vi "testserialRT.vi"() -> ()   [LabVIEW 2017]
uses:
  <vilib>/Instr/_visa.llb/VISA Configure Serial Port (Instr).vi
panel:
  out "error out":errorcluster
  out "s? t:f":i32
  out "4":dbl
  out "3":dbl
  out "2":dbl
  out "1":dbl
  out "Fy":dbl
  out "Fx":dbl
  out "String":string
  in  "stop":bool
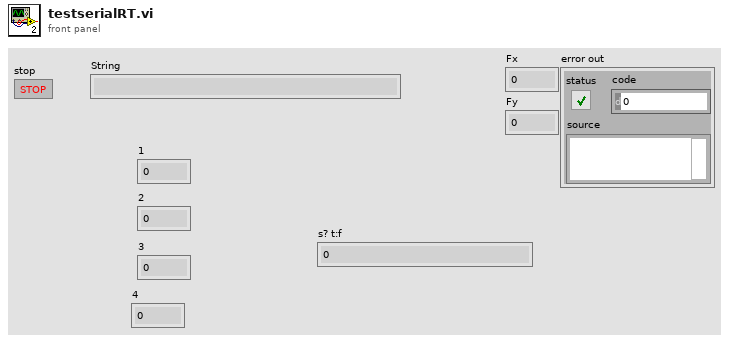
[diagram p1: front panel]
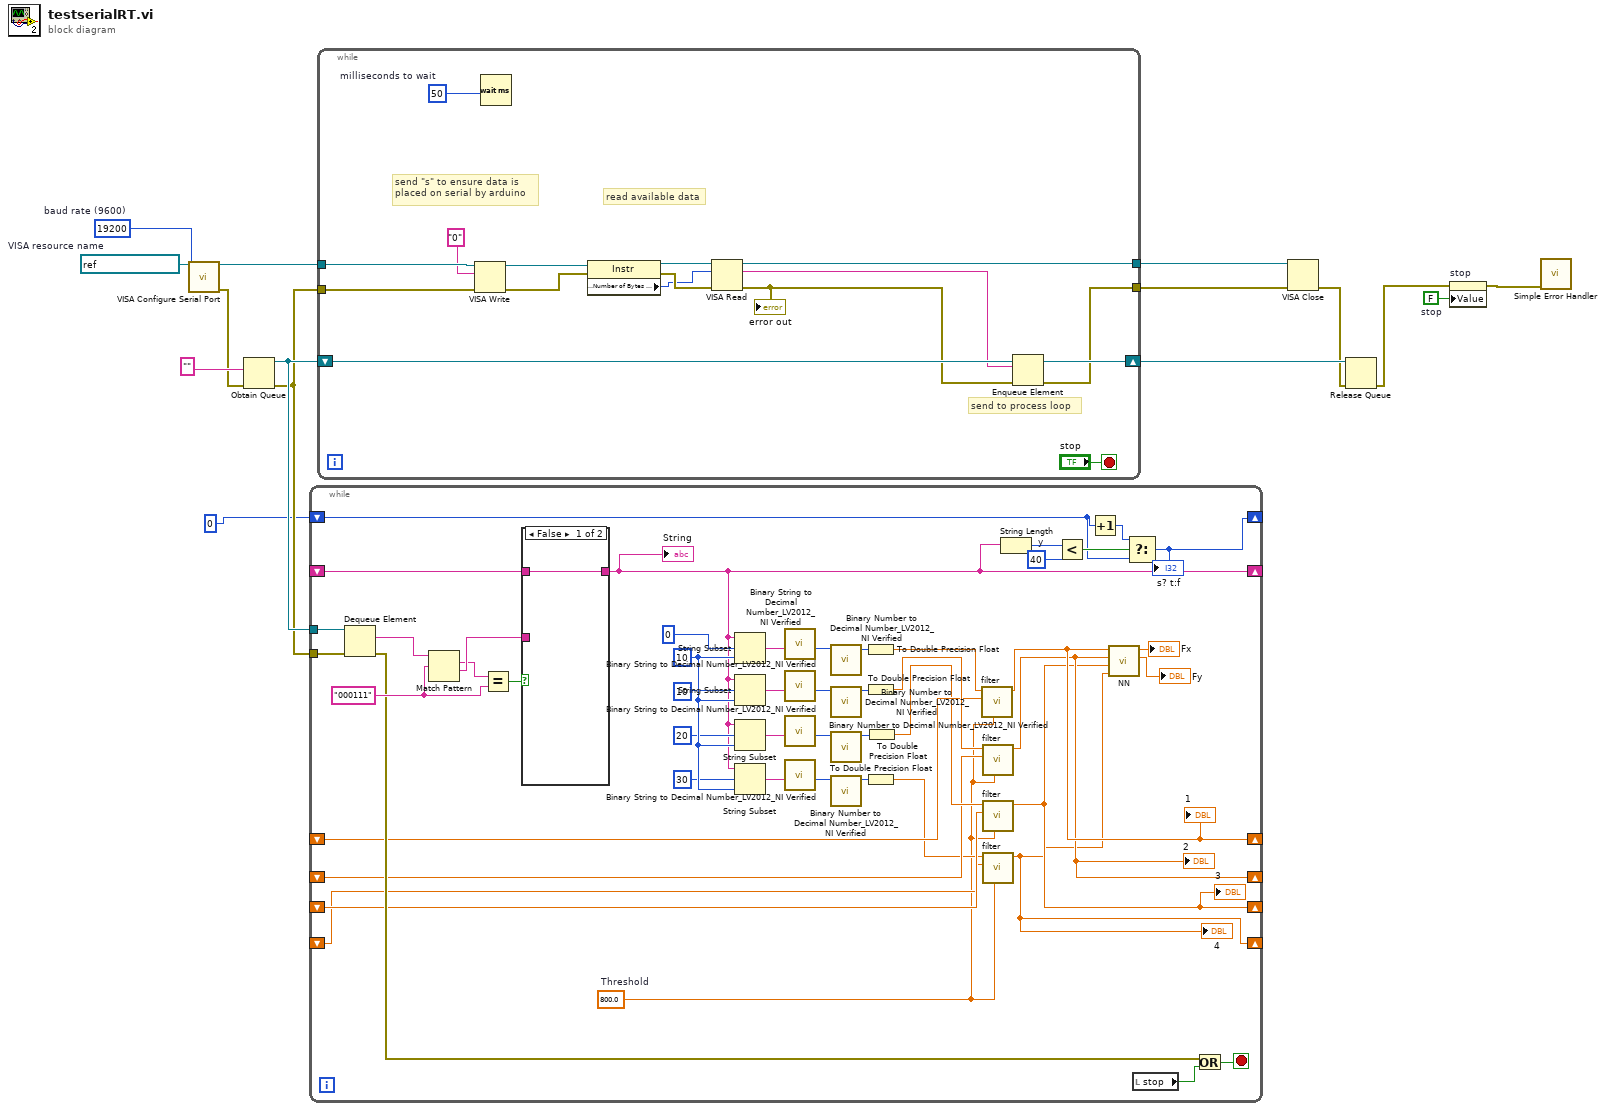
[diagram p0: block diagram]
diagram:
  w1 = u32 19200  # baud rate (9600)
  w3 = FALSE  # stop
  w15 = refnum<visa-resource-name> "ASRL2::INSTR"  # VISA resource name
  n1 = call-poly "VISA Configure Serial Port"("VISA resource name"=w15, "baud rate (9600)"=w1) -> ("VISA resource name out"=w14:refnum<visa-resource-name>, "error out"=w10:errorcluster)  [unwired: 12 in]
  n2 = Obtain Queue(element data type="", error in (no error)=w10) -> (queue out=w7:refnum<queue>, error out=w6:errorcluster)  [unwired: 3 in, 1 out]
  n3 = while {
    tunnel: w7 -> [w65]
    tunnel: w6 -> [w64]
    shift-right: [w22] -> _
    shift-left: _ -> [w56]
    shift-right: [w33] -> _
    shift-left: _ -> [w32]
    shift-right: [w29] -> _
    shift-left: _ -> [w30]
    shift-right: [w28] -> _
    shift-left: _ -> [w27]
    shift-right: [w24] -> _
    shift-left: _ -> [w26]
    shift-right: [w18] -> _
    shift-left: 0 -> [w17]
    stop <- w62 stop-if-true
    w20 = 40  # y
    w23 = 800.0  # Threshold
    w47 = 10 ("length (rest)")
    w58 = "000111" ("y")
    n4 = Dequeue Element(queue=w65, error in (no error)=w64) -> (element=w60:string, error out=w42:errorcluster)  [unwired: 1 in, 2 out]
    n5 = Match Pattern(string=w60, regular expression=w58) -> (match substring=w57:string, after substring=w59:string)  [unwired: 1 in, 2 out]
    n6 = Equal?(x=w57, y=w58) -> (x = y?=w61:bool)
    n7 = case shown="False" w61 {
      tunnel: w59 -> [_ w67]
      tunnel: [w66 w67] -> w22
      tunnel: w56 -> [w66 _]
      frame False {
      }
      frame True {
      }
    }
    "String" <- w22
    n8 = String Subset(string=w22, offset (0)=0, length (rest)=w47) -> (substring=w48:string)
    n9 = String Subset(string=w22, offset (0)=10 ("length (rest)"), length (rest)=w47) -> (substring=w49:string)
    n10 = String Subset(string=w22, offset (0)=20 ("length (rest)"), length (rest)=w47) -> (substring=w50:string)
    n11 = String Subset(string=w22, offset (0)=30 ("length (rest)"), length (rest)=w47) -> (substring=w51:string)
    n12 = call "Binary String to Decimal Number_LV2012_NI Verified.vi"("String"=w48) -> ("Number"=w52:u64)  [unwired: 10 in]
    n13 = call "Binary String to Decimal Number_LV2012_NI Verified.vi"("String"=w49) -> ("Number"=w53:u64)  [unwired: 10 in]
    n14 = call "Binary String to Decimal Number_LV2012_NI Verified.vi"("String"=w50) -> ("Number"=w54:u64)  [unwired: 10 in]
    n15 = call "Binary String to Decimal Number_LV2012_NI Verified.vi"("String"=w51) -> ("Number"=w55:u64)  [unwired: 10 in]
    n16 = call "Binary Number to Decimal Number_LV2012_NI Verified.vi"("Binary number"=w52) -> ("Decimal number"=w41:i64)  [unwired: 10 in]
    n17 = call "Binary Number to Decimal Number_LV2012_NI Verified.vi"("Binary number"=w53) -> ("Decimal number"=w40:i64)  [unwired: 10 in]
    n18 = call "Binary Number to Decimal Number_LV2012_NI Verified.vi"("Binary number"=w54) -> ("Decimal number"=w39:i64)  [unwired: 10 in]
    n19 = call "Binary Number to Decimal Number_LV2012_NI Verified.vi"("Binary number"=w55) -> ("Decimal number"=w38:i64)  [unwired: 10 in]
    n20 = To Double Precision Float(number=w41) -> (double precision float=w35:dbl)
    n21 = To Double Precision Float(number=w40) -> (double precision float=w34:dbl)
    n22 = To Double Precision Float(number=w38) -> (double precision float=w25:dbl)
    n23 = To Double Precision Float(number=w39) -> (double precision float=w31:dbl)
    n24 = call "filter.vi"("Threshold"=w23, "Raw1 old"=w32, "Raw1"=w35) -> ("Raw1 out"=w33:dbl)  [unwired: 8 in]
    "1" <- w33
    n25 = call "filter.vi"("Threshold"=w23, "Raw1 old"=w30, "Raw1"=w34) -> ("Raw1 out"=w29:dbl)  [unwired: 8 in]
    "2" <- w29
    n26 = call "filter.vi"("Threshold"=w23, "Raw1 old"=w27, "Raw1"=w31) -> ("Raw1 out"=w28:dbl)  [unwired: 8 in]
    "3" <- w28
    n27 = call "filter.vi"("Threshold"=w23, "Raw1 old"=w26, "Raw1"=w25) -> ("Raw1 out"=w24:dbl)  [unwired: 8 in]
    "4" <- w24
    n28 = String Length(string=w22) -> (length=w21:i32)
    n29 = Less?(x=w21, y=w20) -> (x < y?=w19:bool)
    n30 = Increment(x=w17) -> (x+1=w16:i32)
    n31 = call "NN.vi"("Raw4"=w24, "Raw3"=w28, "Raw2"=w29, "Raw1"=w33) -> ("Fy"=→"Fy":dbl, "Fx"=→"Fx":dbl)  [unwired: 6 in]
    n32 = Select(t=w16, s=w19, f=w17) -> (s? t:f=w18:i32)
    "s? t:f" <- w18
    n33 = local read "stop"() -> (w63:bool)
    n34 = Or(x=w42, y=w63) -> (x .or. y?=w62:bool)
  }
  n35 = while {
    tunnel: w14 -> [w82]
    tunnel: w6 -> [w81]
    tunnel: [w69] -> w13
    tunnel: [w77] -> w12
    shift-right: [w80] -> w9
    shift-left: w7 -> [w78]
    stop <- "stop" stop-if-true
    w79 = u32 50  # milliseconds to wait
    # "send to process loop"
    # "read available data"
    # "send \"s\" to ensure data is\nplaced on serial by arduino"
    n36 = VISA Write(VISA resource name=w82, write buffer="0", error in (no error)=w81) -> (VISA resource name out=w71:refnum<visa-resource-name>, error out=w70:errorcluster)  [unwired: 1 out]
    n37 = Wait (ms)(milliseconds to wait=w79) -> ()  [unwired: 1 out]
    n38 = property class="Instr"(reference=w71, error in=w70) -> (reference out=w75:refnum<visa-resource-name>, error out=w74:errorcluster, "Serial Settings:Number of Bytes at Serial Port"=w73:u32)
    n39 = VISA Read(VISA resource name=w75, byte count=w73, error in (no error)=w74) -> (VISA resource name out=w69:refnum<visa-resource-name>, read buffer=w76:string, error out=w68:errorcluster)  [unwired: 1 out]
    "error out" <- w68
    n40 = Enqueue Element(queue=w78, element=w76, error in (no error)=w68) -> (queue out=w80:refnum<queue>, error out=w77:errorcluster)  [unwired: 1 in, 1 out]
  }
  n41 = VISA Close(VISA resource name=w13, error in (no error)=w12) -> (error out=w8:errorcluster)
  n42 = Release Queue(queue=w9, error in (no error)=w8) -> (error out=w5:errorcluster)  [unwired: 1 in, 2 out]
  n43 = property on="stop" class="Bool (strict)"(error in=w5, "Value"=w3) -> (error out=w4:errorcluster)  [unwired: 1 in, 1 out]
  n44 = call <vilib>:"Simple Error Handler.vi"("error in (no error)"=w4) -> ()  [unwired: 4 in, 5 out]
